vi "Setup.vi"(8 "error in (no error)":errorcluster) -> (0 "error out":errorcluster, 3 "1553 Unit Test out":refnum<class "Remote Terminal.lvclass">)   [LabVIEW 2020, in "Unit Tests.lvlib" / "Remote Terminal.lvclass"]
uses:
  Remote Terminal.lvclass
  Remote Terminal.lvclass/Remote Terminal.ctl
  Utilities/Simulated FPGA/FPGA Sim.lvclass
  C:/Users/MattJ/Desktop/git/bci-1553-labview-api/src/Dependencies/FPGA Interface/FPGA Interface.lvclass
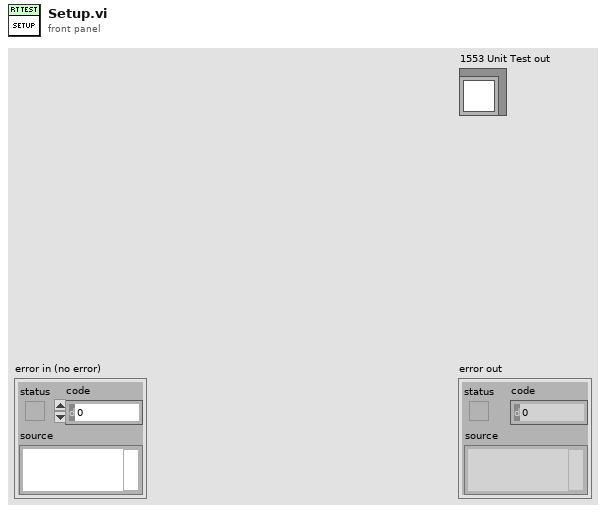
[diagram p1: front panel]
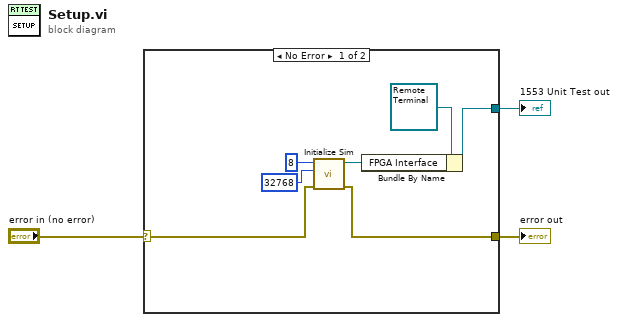
[diagram p0: block diagram]
diagram:
  n1 = case shown="No Error" "error in (no error)" {
    selector: "error in (no error)" -> [w5 w11]
    tunnel: [w4 w11] -> w2
    tunnel: [w9 _] -> w1
    frame No Error {
      n2 = call "Initialize Sim.vi"("error in (no error)"=w5, "Memory Size (32k)"=32768, "Components (8)"=8) -> ("error out"=w4:errorcluster, "FPGA Sim out"=w8:refnum<class "FPGA Sim.lvclass">)  [unwired: 7 in]
      n3 = Bundle By Name(cluster=refnum<class "Remote Terminal.lvclass"> refnum ("Remote Terminal in"), "FPGA Interface"=w8) -> (w9:refnum<class "Remote Terminal.lvclass">)
    }
    frame Error {
    }
  }
  "error out" <- w2
  "1553 Unit Test out" <- w1
